vi "Grid_adjustZ.vi"(8 "error in":errorcluster, 9 "FileRefs":T2, 10 "Settings":T1={"Drift Correction Settings"={"Drift Correction every"=80, "Drift correction Pixels"=256, "Channel index (0-23)"=0, "MaxImagesBack"=2, "Threshold"=2, "Increment"=8, "max applied Drift Correction"=20, "Correct Drift"=TRUE, "Correlate"=0, "Correct z drift"=FALSE, "zdrift \nDuration (s)"=0.0}, "Spectroscopy Setting"={"Imaging Current"=1e-11, "ref Current"=7e-11, "tip Speed (m/s)"=2e-09, "Imaging Bias"=0.02, "ref Bias"=-0.1, "preSTS delay [ms]"=500, "STS z offset"=2e-10, "during Spec Bias (V)"=-0.1, "trigger1 < Hz"=0.0, "trigger 2 >Hz"=0.0, "autoStop"=FALSE, "Spectroscopy"=0, "PLL ON/OFF"=TRUE, "readjust setpoint every "=1, "z Reference"=FALSE, "Lock In"=TRUE}, "Misc"={"File name"="symmetric_node_zOff=200p", "Email when finished"="cornelius.krull@monash.edu,Dhaneesh.Gopalakrishnan@monash.edu,marina.castelli@monash.edu"}, "Grid Settings"={"type"=1, "type order"=1, "X pixel"=0, "Y pixel"=0, "Grid_Parms"={"center X (m)"=0.0, "center Y (m)"=0.0, "width (m)"=0.0, "height (m)"=0.0, "angle (deg)"=0.0}}} {"Grid Settings"."type order" items=["Line", "Grid"]; "Grid Settings"."type" items=["Line", "Grid"]; "Spectroscopy Setting"."Spectroscopy" items=["Bias", "zSpec"]; "Spectroscopy Setting"."trigger 2 >Hz" format="%#_6p"; "Spectroscopy Setting"."trigger1 < Hz" format="%#_6p"; "Spectroscopy Setting"."during Spec Bias (V)" format="%#_5p"; "Spectroscopy Setting"."STS z offset" format="%#_6p"; "Spectroscopy Setting"."ref Bias" format="%#_6p"; "Spectroscopy Setting"."Imaging Bias" format="%#_6p"; "Spectroscopy Setting"."tip Speed (m/s)" format="%.2p"; "Spectroscopy Setting"."ref Current" format="%#_6p"; "Spectroscopy Setting"."Imaging Current" format="%#_6p"; "Drift Correction Settings"."Correlate" items=["first Frame", "successive Frames"]; "Drift Correction Settings"."max applied Drift Correction" min=1 max=100 step=1 format="%.0p"; "Drift Correction Settings"."Threshold" min=1 step=1; "Drift Correction Settings"."Channel index (0-23)" items=["Current"=0, "Z (m)"=14]}, 11 "Application in":refnum<vi>) -> (0 "error out":errorcluster, 1 "FileRefs out":T2, 2 "Settings out":T1={"Drift Correction Settings"={"Drift Correction every"=80, "Drift correction Pixels"=256, "Channel index (0-23)"=0, "MaxImagesBack"=2, "Threshold"=2, "Increment"=8, "max applied Drift Correction"=20, "Correct Drift"=TRUE, "Correlate"=0, "Correct z drift"=FALSE, "zdrift \nDuration (s)"=0.0}, "Spectroscopy Setting"={"Imaging Current"=1e-11, "ref Current"=7e-11, "tip Speed (m/s)"=2e-09, "Imaging Bias"=0.02, "ref Bias"=-0.1, "preSTS delay [ms]"=500, "STS z offset"=2e-10, "during Spec Bias (V)"=-0.1, "trigger1 < Hz"=0.0, "trigger 2 >Hz"=0.0, "autoStop"=FALSE, "Spectroscopy"=0, "PLL ON/OFF"=TRUE, "readjust setpoint every "=1, "z Reference"=FALSE, "Lock In"=TRUE}, "Misc"={"File name"="symmetric_node_zOff=200p", "Email when finished"="cornelius.krull@monash.edu,Dhaneesh.Gopalakrishnan@monash.edu,marina.castelli@monash.edu"}, "Grid Settings"={"type"=1, "type order"=1, "X pixel"=0, "Y pixel"=0, "Grid_Parms"={"center X (m)"=0.0, "center Y (m)"=0.0, "width (m)"=0.0, "height (m)"=0.0, "angle (deg)"=0.0}}} {"Grid Settings"."type order" items=["Line", "Grid"]; "Grid Settings"."type" items=["Line", "Grid"]; "Spectroscopy Setting"."Spectroscopy" items=["Bias", "zSpec"]; "Spectroscopy Setting"."trigger 2 >Hz" format="%#_6p"; "Spectroscopy Setting"."trigger1 < Hz" format="%#_6p"; "Spectroscopy Setting"."during Spec Bias (V)" format="%#_5p"; "Spectroscopy Setting"."STS z offset" format="%#_6p"; "Spectroscopy Setting"."ref Bias" format="%#_6p"; "Spectroscopy Setting"."Imaging Bias" format="%#_6p"; "Spectroscopy Setting"."tip Speed (m/s)" format="%.2p"; "Spectroscopy Setting"."ref Current" format="%#_6p"; "Spectroscopy Setting"."Imaging Current" format="%#_6p"; "Drift Correction Settings"."Correlate" items=["first Frame", "successive Frames"]; "Drift Correction Settings"."max applied Drift Correction" min=1 max=100 step=1 format="%.0p"; "Drift Correction Settings"."Threshold" min=1 step=1; "Drift Correction Settings"."Channel index (0-23)" items=["Current"=0, "Z (m)"=14]}, 3 "Application ref out":refnum<vi>, 5 "Last z adjustment":dbl)   [LabVIEW 2021]
uses:
  <userlib>/Nanonis Prog Interface V5/Nanonis Prog Interface.lvlib
panel:
  # "z Spectroscopy"
  # "GRID points"
  # "Increase this if no Drift was detected for \na certain number of images"
  # "% of image size"
  # "z Spectroscopy"
  # "GRID points"
  # "Increase this if no Drift was detected for \na certain number of images"
  # "% of image size"
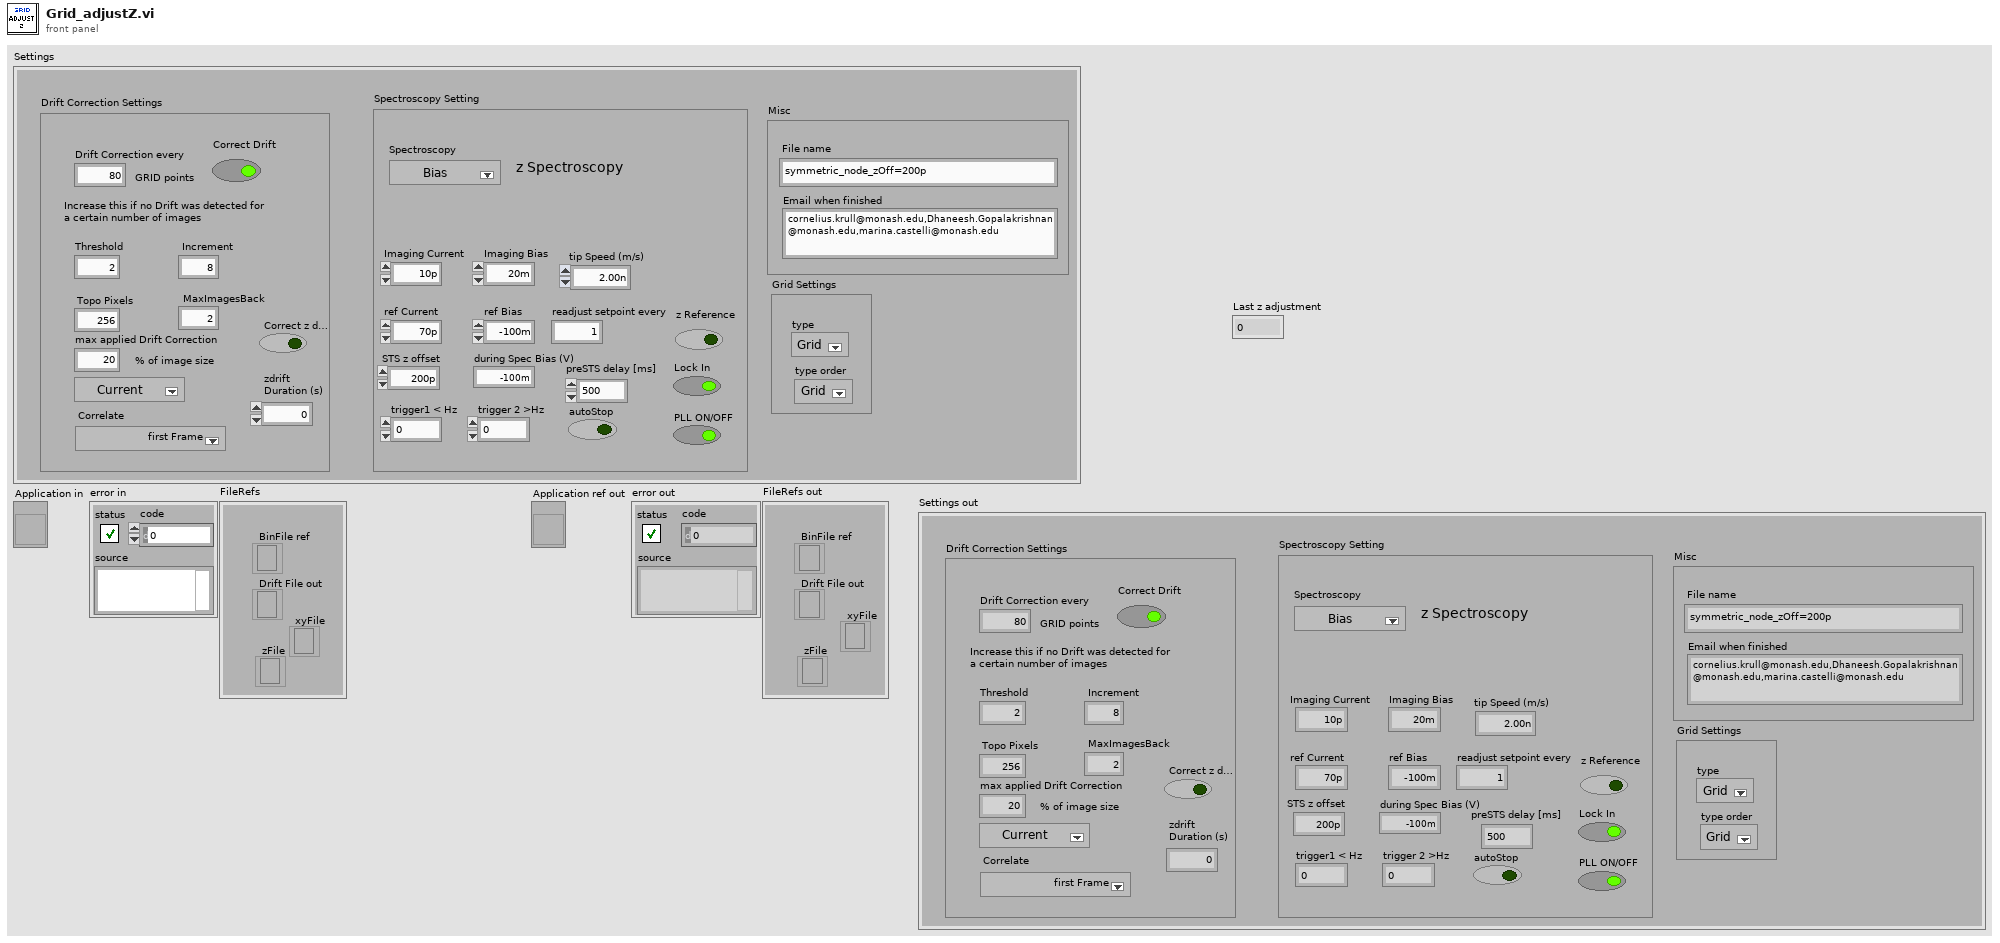
[diagram p1: front panel]
types:
  T1 = cluster{"Drift Correction Settings":cluster{"Drift Correction every":i32, "Drift correction Pixels":i32, "Channel index (0-23)":u8, "MaxImagesBack":i32, "Threshold":i32, "Increment":i32, "max applied Drift Correction":i32, "Correct Drift":bool, "Correlate":u16, "Correct z drift":bool, "zdrift \nDuration (s)":dbl}, "Spectroscopy Setting":cluster{"Imaging Current":dbl, "ref Current":dbl, "tip Speed (m/s)":sgl, "Imaging Bias":dbl, "ref Bias":dbl, "preSTS delay [ms]":u32, "STS z offset":dbl, "during Spec Bias (V)":sgl, "trigger1 < Hz":sgl, "trigger 2 >Hz":sgl, "autoStop":bool, "Spectroscopy":u16, "PLL ON/OFF":bool, "readjust setpoint every ":i32, "z Reference":bool, "Lock In":bool}, "Misc":cluster{"File name":string, "Email when finished":string}, "Grid Settings":cluster{"type":u16, "type order":u16, "X pixel":i32, "Y pixel":i32, "Grid_Parms":cluster{"center X (m)":sgl, "center Y (m)":sgl, "width (m)":sgl, "height (m)":sgl, "angle (deg)":sgl}}}
  T2 = cluster{"Drift File out":refnum<file>, "zFile":refnum<file>, "BinFile ref":refnum<file>, "xyFile":refnum<file>}
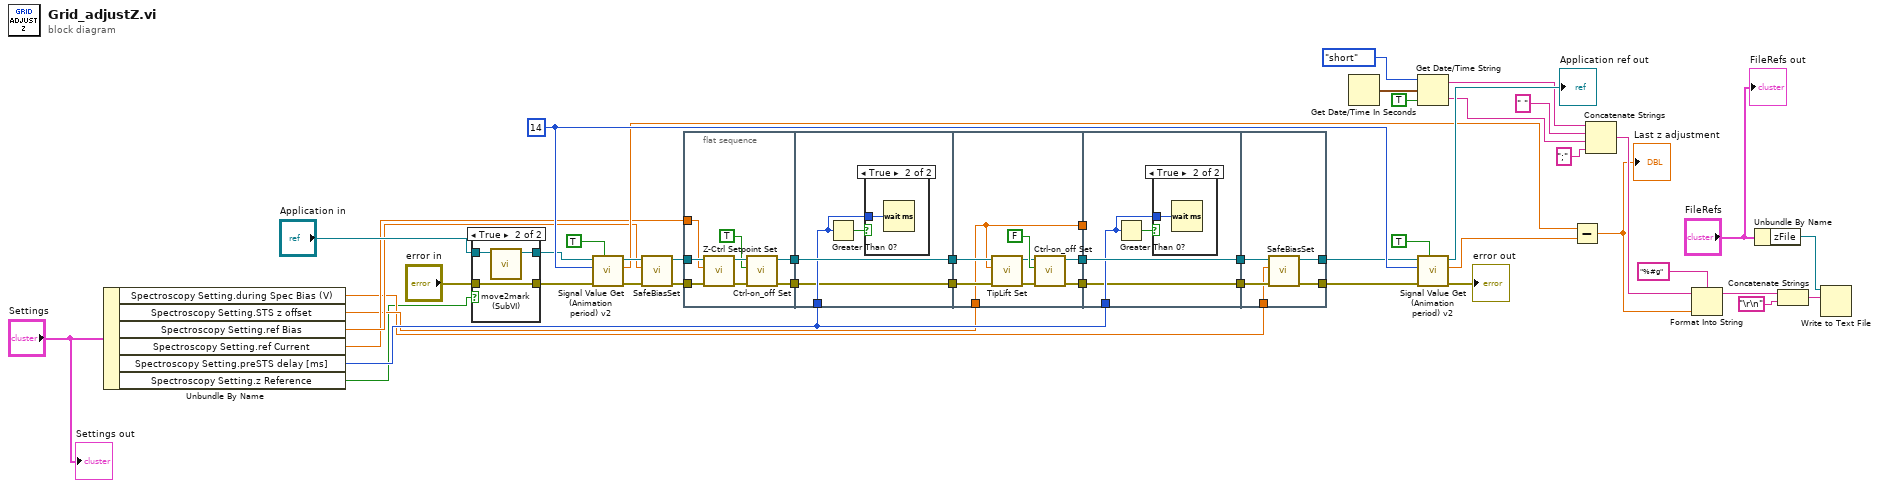
[diagram p0: block diagram]
diagram:
  w47 = 14 ("index of element")
  n1 = Unbundle By Name("Settings") -> ("Spectroscopy Setting.during Spec Bias (V)"=w9:sgl, "Spectroscopy Setting.STS z offset"=w10:dbl, "Spectroscopy Setting.ref Bias"=w13:dbl, "Spectroscopy Setting.ref Current"=w12:dbl, "Spectroscopy Setting.preSTS delay [ms]"=w14:u32, "Spectroscopy Setting.z Reference"=w7:bool)
  n2 = case shown="True" w7 {
    tunnel: "Application in" -> [w50 w53]
    tunnel: [w50 w52] -> w36
    tunnel: "error in" -> [w49 w51]
    tunnel: [w49 w51] -> w1
    frame False {
    }
    frame True {
      n3 = call "move2mark (SubVI).vi"("Application in"=w53) -> ("Application out"=w52:refnum<vi>)  [unwired: 10 in]
    }
  }
  n4 = call <userlib>:"Signal Value Get (Animation period) v2.vi"("Wait for newest data (F=False)"=TRUE, "error in (no error)"=w1, "Signal index (0-79)"=w47, "Application ref in"=w36) -> ("error out"=w19:errorcluster, "Signal value"=w30:sgl, "Application ref out"=w35:refnum<vi>)  [unwired: 4 in]
  n5 = call "SafeBiasSet.vi"("Application ref in"=w35, "Bias (V)"=w13, "error in (no error)"=w19) -> ("Application ref out"=w37:refnum<vi>, "Error out"=w18:errorcluster)  [unwired: 6 in]
  n6 = flat-sequence {
    tunnel: w37 -> [w61]
    tunnel: [w58] -> w46
    tunnel: w12 -> [w60]
    tunnel: w18 -> [w56]
    tunnel: [w54] -> w45
    tunnel: w46 -> [w65]
    tunnel: [w65] -> w44
    tunnel: w14 -> [w63]
    tunnel: [w62] -> w43
    tunnel: w45 -> [w62]
    tunnel: w44 -> [w73]
    tunnel: [w71] -> w42
    tunnel: [w67] -> w41
    tunnel: w43 -> [w70]
    tunnel: [w68] -> w40
    tunnel: w10 -> [w67]
    tunnel: w42 -> [w78]
    tunnel: w14 -> [w77]
    tunnel: w41 -> [_]
    tunnel: [w78] -> w39
    tunnel: [w75] -> w38
    tunnel: w40 -> [w75]
    tunnel: [w83] -> w33
    tunnel: w39 -> [w84]
    tunnel: w38 -> [w82]
    tunnel: [w81] -> w17
    tunnel: w9 -> [w80]
    frame #0 {
      n7 = call <userlib>:"Z-Ctrl Setpoint Set.vi"("error in (no error)"=w56, "Z Controller setpoint"=w60, "Application ref in"=w61) -> ("error out"=w55:errorcluster, "Application ref out"=w59:refnum<vi>)  [unwired: 7 in]
      n8 = call <userlib>:"Ctrl-on_off Set.vi"("error in (no error)"=w55, "Z Controller ON/OFF"=TRUE, "Application ref in"=w59) -> ("error out"=w54:errorcluster, "Application ref out"=w58:refnum<vi>)  [unwired: 7 in]
    }
    frame #1 {
      n9 = Greater Than 0?(x=w63) -> (x > 0?=w64:bool)
      n10 = case shown="True" w64 {
        tunnel: w63 -> [_ w66]
        frame False {
        }
        frame True {
          n11 = Wait (ms)(milliseconds to wait=w66) -> ()  [unwired: 1 out]
        }
      }
    }
    frame #2 {
      n12 = call <userlib>:"TipLift Set.vi"("error in (no error)"=w70, "TipLift (m)"=w67, "Application ref in"=w73) -> ("error out"=w69:errorcluster, "Application ref out"=w72:refnum<vi>)  [unwired: 7 in]
      n13 = call <userlib>:"Ctrl-on_off Set.vi"("error in (no error)"=w69, "Z Controller ON/OFF"=FALSE, "Application ref in"=w72) -> ("error out"=w68:errorcluster, "Application ref out"=w71:refnum<vi>)  [unwired: 7 in]
    }
    frame #3 {
      n14 = Greater Than 0?(x=w77) -> (x > 0?=w76:bool)
      n15 = case shown="True" w76 {
        tunnel: w77 -> [_ w79]
        frame False {
        }
        frame True {
          n16 = Wait (ms)(milliseconds to wait=w79) -> ()  [unwired: 1 out]
        }
      }
    }
    frame #4 {
      n17 = call "SafeBiasSet.vi"("Application ref in"=w84, "Bias (V)"=w80, "error in (no error)"=w82) -> ("Application ref out"=w83:refnum<vi>, "Error out"=w81:errorcluster)  [unwired: 6 in]
    }
  }
  n18 = Get Date/Time In Seconds() -> (seconds since 1Jan1904=w24:timestamp)
  n19 = Get Date/Time String(date format (0)=enum16{"short", "long", "abbreviated"}."short", seconds (now)=w24, want seconds? (F)=TRUE) -> (date string=w4:string, time string=w27:string)
  n20 = call <userlib>:"Signal Value Get (Animation period) v2.vi"("Wait for newest data (F=False)"=TRUE, "error in (no error)"=w17, "Signal index (0-79)"=w47, "Application ref in"=w33) -> ("error out"=→"error out":errorcluster, "Signal value"=w29:sgl, "Application ref out"=→"Application ref out":refnum<vi>)  [unwired: 4 in]
  n21 = Subtract(x=w30, y=w29) -> (x-y=w8:sgl)
  "Last z adjustment" <- w8
  n22 = Concatenate Strings(w4, " " ("string"), w27, ";" ("string")) -> (w26:string)
  n23 = Format Into String(format string="%#g", initial string=w26, w8) -> (resulting string=w21:string)  [unwired: 1 in, 1 out]
  n24 = Unbundle By Name("FileRefs") -> ("zFile"=w6:refnum<file>)
  n25 = Concatenate Strings(w21, "\r\n") -> (w5:string)
  n26 = Write to Text File(file (use dialog)=w6, text=w5) -> ()  [unwired: 2 in, 3 out]
  "FileRefs out" <- "FileRefs"
  "Settings out" <- "Settings"
